vi "Poll.vi"(8 "error in":errorcluster, 11 "VISA resource name in":refnum<visa-resource-name>) -> (0 "error out":errorcluster, 2 "Read":string, 3 "VISA resource name out":refnum<visa-resource-name>)   [LabVIEW 2015]
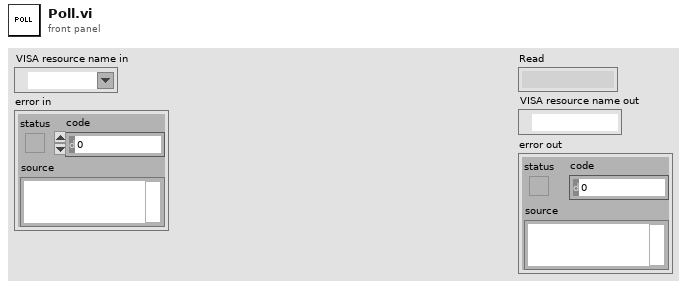
[diagram p1: front panel]
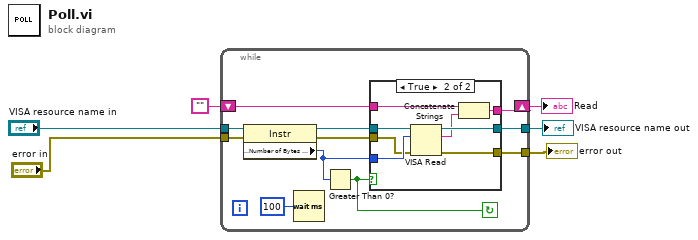
[diagram p0: block diagram]
diagram:
  n1 = while {
    tunnel: [w13] -> w2
    tunnel: "VISA resource name in" -> [w12]
    tunnel: "error in" -> [w11]
    shift-right: [w10] -> w3
    shift-left: "" -> [w9]
    tunnel: [w8] -> w1
    stop <- w17 continue-if-true
    n2 = property class="Instr"(reference=w12, error in=w11) -> (reference out=w16:refnum<visa-resource-name>, error out=w15:errorcluster, "Serial Settings:Number of Bytes at Serial Port"=w14:u32)
    n3 = Wait (ms)(milliseconds to wait=u32 100) -> ()  [unwired: 1 out]
    n4 = Greater Than 0?(x=w14) -> (x > 0?=w17:bool)
    n5 = case shown="True" w17 {
      tunnel: w16 -> [w20 w28]
      tunnel: w15 -> [w18 w26]
      tunnel: w14 -> [_ w27]
      tunnel: [w20 w25] -> w13
      tunnel: [w19 w23] -> w10
      tunnel: w9 -> [w19 w22]
      tunnel: [w18 w21] -> w8
      frame False {
      }
      frame True {
        n6 = VISA Read(VISA resource name=w28, byte count=w27, error in (no error)=w26) -> (VISA resource name out=w25:refnum<visa-resource-name>, read buffer=w24:string, error out=w21:errorcluster)  [unwired: 1 out]
        n7 = Concatenate Strings(w22, w24) -> (w23:string)
      }
    }
  }
  "Read" <- w3
  "VISA resource name out" <- w2
  "error out" <- w1
